vi "Extract Send.vi"(7 "Copy":bool caption="Copy data instead of extracting", 8 "error in (no error)":errorcluster, 11 "Message(Send) in":refnum<class "MSG.lvclass">) -> (0 "error out":errorcluster, 1 "Send Object":refnum<class "Send.lvclass">, 2 "Label":string, 3 "Message(Send) out":refnum<class "MSG.lvclass">)   [LabVIEW 2011, in "Messenging.lvlib" / "MSG.lvclass"]
uses:
  MSG.lvclass
  Send/Send.lvclass
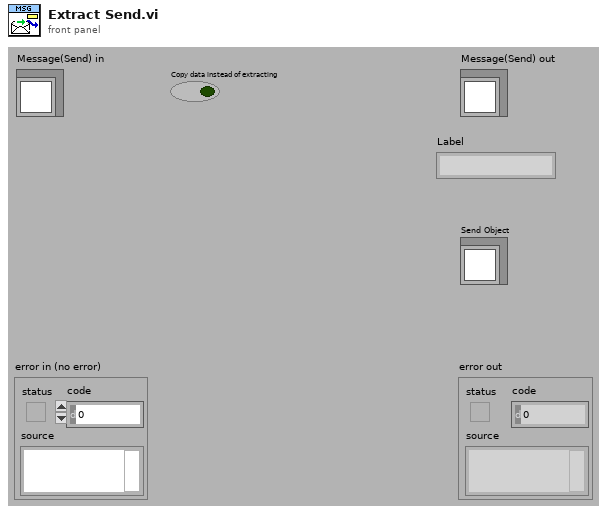
[diagram p1: front panel]
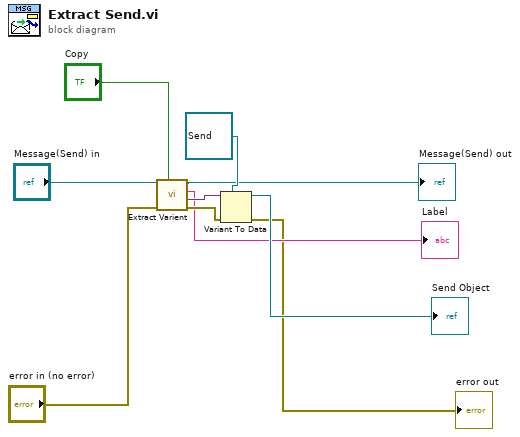
[diagram p0: block diagram]
diagram:
  n1 = call-dynamic "Extract Varient.vi"("Copy"="Copy", "error in (no error)"="error in (no error)", "Message"="Message(Send) in") -> ("error out"=w9:errorcluster, "Varient"=w10:variant, "Label"=→"Label":string, "Message"=→"Message(Send) out":refnum<class "MSG.lvclass">)  [unwired: 5 out]
  n2 = Variant To Data(error in=w9, type=refnum<class "Send.lvclass"> refnum ("MSR Parent in"), Variant=w10) -> (data=→"Send Object":refnum<class "Send.lvclass">, error out=→"error out":errorcluster)
